vi "Custom Drive Motors.vi"(8 "error in (no error)":errorcluster, 9 "RightSpeed":dbl, 10 "LeftSpeed":dbl, 11 "RobotDriveDevRef":T1={"DevStatus"={"status"=FALSE, "code"=0, "source"=""}, "Motors[]"=[], "Square Inputs"=FALSE, "Max Output"=1.0}) -> (0 "error out":errorcluster, 2 "Motor Values":dbl[](array[numeric]), 3 "RobotDriveDevRef":T1={"DevStatus"={"status"=FALSE, "code"=0, "source"=""}, "Motors[]"=[], "Square Inputs"=FALSE, "Max Output"=1.0})   [LabVIEW 2015]
doc: "Determines the motor configuration and sends the speed values to the appropriate motors.\n\nThis software is licensed. Open the labview\\readme\\WPI Robotics Library Open Source License.txt file for more information."
uses:
  <vilib>/Rock Robotics/WPI/RobotDrive/WPI_RobotDriveDevRef.ctl
  <vilib>/Rock Robotics/WPI/MotorControl/WPI_MotorControlDeviceRef.ctl
  <vilib>/Rock Robotics/WPI/MotorControl/WPI_MotorControlType.ctl
  <vilib>/Rock Robotics/SystemInterfaces/DIO/FPGA_DIOPWMChannel.ctl
  <vilib>/Rock Robotics/WPI/PWM/WPI_PWMDeadband.ctl
  <vilib>/Rock Robotics/WPI/CAN/Jaguar/SubVIs/WPI_CANJaguar_ControlMode.ctl
  <vilib>/Rock Robotics/WPI/CAN/TalonSRX/WPI_CANTalonSRX_APIControlMode.ctl
  <vilib>/Rock Robotics/WPI/RobotDrive/WPI_RobotDriveSafetyCheck.vi
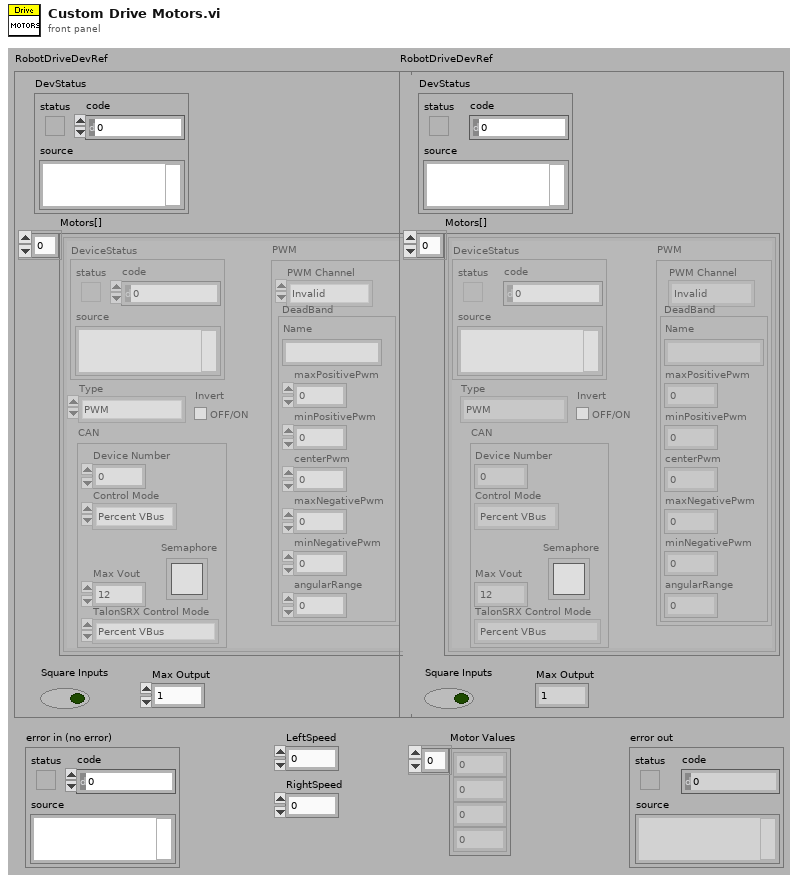
[diagram p1: front panel]
types:
  T1 = typedef "WPI_RobotDriveDevRef.ctl" = cluster{"DevStatus":errorcluster, "Motors[]":T2[], "Square Inputs":bool, "Max Output":dbl}
  T2 = typedef "WPI_MotorControlDeviceRef.ctl" = cluster{"DeviceStatus":errorcluster, "Type":T3, "PWM":cluster{"PWM Channel":T4, "DeadBand":T5}, "CAN":cluster{"Device Number":u8, "Control Mode":T6, "Semaphore":T7, "Max Vout":dbl, "TalonSRX Control Mode":T8}, "Invert":bool}
  T3 = typedef "WPI_MotorControlType.ctl" = enum16{"PWM", "CAN", "CANTalonSRX"}
  T4 = typedef "FPGA_DIOPWMChannel.ctl" = enum8{"PWM 0", "PWM 1", "PWM 2", "PWM 3", "PWM 4", "PWM 5", "PWM 6", "PWM 7", "PWM 8", "PWM 9", "PWM MXP 0", "PWM MXP 1", "PWM MXP 2", "PWM MXP 3", "PWM MXP 4", "PWM MXP 5", "PWM MXP 6", "PWM MXP 7", "PWM MXP 8", "PWM MXP 9", "Invalid"}
  T5 = typedef "WPI_PWMDeadband.ctl" = cluster{"Name":string, "maxPositivePwm":i32, "minPositivePwm":i32, "centerPwm":i32, "maxNegativePwm":i32, "minNegativePwm":i32, "angularRange":u16}
  T6 = typedef "WPI_CANJaguar_ControlMode.ctl" = enum8{"Percent VBus", "Current", "Speed", "Position", "Voltage"}
  T7 = typedef "Semaphore RefNum" = refnum<k1>
  T8 = typedef "WPI_CANTalonSRX_APIControlMode.ctl" = enum8{"Percent VBus", "Speed", "Position", "Slave", "Unchanged / Invalid", "Voltage Compensation", "Current", "Motion Profile"}
  T9 = enum16{"Rear Left Motor", "Rear Right Motor", "Front Left Motor", "Front Right Motor", "Middle Right Motor", "Middle Left Motor"}
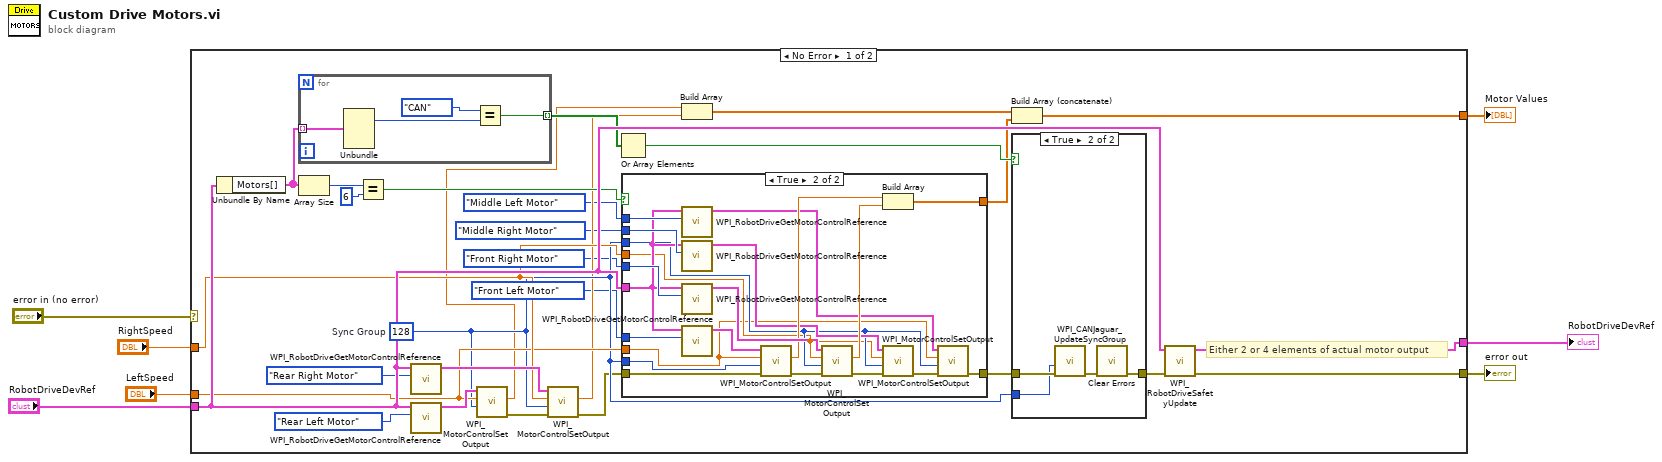
[diagram p0: block diagram]
diagram:
  n1 = case shown="No Error" "error in (no error)" {
    selector: "error in (no error)" -> [_ w69]
    tunnel: "RobotDriveDevRef" -> [w32 w68]
    tunnel: [w14 w68] -> w6
    tunnel: "LeftSpeed" -> [w30 _]
    tunnel: "RightSpeed" -> [w31 _]
    tunnel: [w15 w69] -> w2
    tunnel: [w17 _] -> w1
    frame No Error {
      w28 = u8 128  # Sync Group
      # "Either 2 or 4 elements of actual motor output"
      n2 = Unbundle By Name(w32) -> ("Motors[]"=w27:T2[])
      n3 = for {
        tunnel: w27 -> [w40] mode=indexing
        tunnel: [w37] -> w26 mode=indexing
        n4 = Unbundle(w40) -> ("Type"=w39:T3)  [unwired: 4 out]
        n5 = Equal?(x=enum16{"PWM", "CAN"}."CAN" ("Type"), y=w39) -> (x = y?=w37:bool)
      }
      n6 = Array Size(array=w27) -> (size(s)=w36:i32)
      n7 = Equal?(x=w36, y=6) -> (x = y?=w29:bool)
      n8 = call <vilib>:"WPI_RobotDriveGetMotorControlReference.vi"("MotorIndex"=T9."Rear Right Motor", "RobotDriveDevRef"=w32) -> ("MotorControlDeviceRef"=w34:T2)  [unwired: 9 out]
      n9 = call <vilib>:"WPI_RobotDriveGetMotorControlReference.vi"("MotorIndex"=T9."Rear Left Motor", "RobotDriveDevRef"=w32) -> ("MotorControlDeviceRef"=w33:T2)  [unwired: 9 out]
      n10 = call <vilib>:"WPI_MotorControlSetOutput.vi"("Sync Group / Parameter Slot"=w28, "Output"=w30, "MotorControlDevRef"=w33) -> ("error out"=w24:errorcluster, "Motor Output"=w21:dbl)  [unwired: 2 in, 5 out]
      n11 = call <vilib>:"WPI_MotorControlSetOutput.vi"("error in (no error)"=w24, "Sync Group / Parameter Slot"=w28, "Output"=w31, "MotorControlDevRef"=w34) -> ("error out"=w22:errorcluster, "Motor Output"=w20:dbl)  [unwired: 1 in, 5 out]
      n12 = Or Array Elements(Boolean array=w26) -> (logical OR=w25:bool)
      n13 = case shown="True" w29 {
        tunnel: T9."Front Left Motor" -> [_ w67]
        tunnel: T9."Front Right Motor" -> [_ w66]
        tunnel: w32 -> [_ w53]
        tunnel: w28 -> [_ w52]
        tunnel: w31 -> [_ w51]
        tunnel: w30 -> [_ w50]
        tunnel: [w46 w47] -> w23
        tunnel: w28 -> [_ w63]
        tunnel: w22 -> [w46 w61]
        tunnel: [_ w58] -> w19
        tunnel: T9."Middle Right Motor" -> [_ w56]
        tunnel: T9."Middle Left Motor" -> [_ w55]
        frame False {
        }
        frame True {
          n14 = call <vilib>:"WPI_RobotDriveGetMotorControlReference.vi"("MotorIndex"=w55, "RobotDriveDevRef"=w53) -> ("MotorControlDeviceRef"=w54:T2)  [unwired: 9 out]
          n15 = call <vilib>:"WPI_RobotDriveGetMotorControlReference.vi"("MotorIndex"=w56, "RobotDriveDevRef"=w53) -> ("MotorControlDeviceRef"=w57:T2)  [unwired: 9 out]
          n16 = call <vilib>:"WPI_RobotDriveGetMotorControlReference.vi"("MotorIndex"=w66, "RobotDriveDevRef"=w53) -> ("MotorControlDeviceRef"=w65:T2)  [unwired: 9 out]
          n17 = call <vilib>:"WPI_RobotDriveGetMotorControlReference.vi"("MotorIndex"=w67, "RobotDriveDevRef"=w53) -> ("MotorControlDeviceRef"=w64:T2)  [unwired: 9 out]
          n18 = call <vilib>:"WPI_MotorControlSetOutput.vi"("error in (no error)"=w61, "Sync Group / Parameter Slot"=w63, "Output"=w50, "MotorControlDevRef"=w64) -> ("error out"=w62:errorcluster, "Motor Output"=w59:dbl)  [unwired: 1 in, 5 out]
          n19 = call <vilib>:"WPI_MotorControlSetOutput.vi"("error in (no error)"=w62, "Sync Group / Parameter Slot"=w52, "Output"=w51, "MotorControlDevRef"=w65) -> ("error out"=w49:errorcluster, "Motor Output"=w60:dbl)  [unwired: 1 in, 5 out]
          n20 = Build Array(w59, w60) -> (w58:dbl[])
          n21 = call <vilib>:"WPI_MotorControlSetOutput.vi"("error in (no error)"=w49, "Sync Group / Parameter Slot"=w52, "Output"=w51, "MotorControlDevRef"=w57) -> ("error out"=w48:errorcluster)  [unwired: 1 in, 6 out]
          n22 = call <vilib>:"WPI_MotorControlSetOutput.vi"("error in (no error)"=w48, "Sync Group / Parameter Slot"=w52, "Output"=w50, "MotorControlDevRef"=w54) -> ("error out"=w47:errorcluster)  [unwired: 1 in, 6 out]
        }
      }
      n23 = Build Array(w21, w20) -> (w18:dbl[])
      n24 = Build Array (concatenate)(w18, w19) -> (w17:dbl[])
      n25 = case shown="True" w25 {
        tunnel: w23 -> [w41 w44]
        tunnel: w28 -> [_ w43]
        tunnel: [w41 w42] -> w16
        frame False {
        }
        frame True {
          n26 = call <vilib>:"WPI_CANJaguar_UpdateSyncGroup.vi"("error in (no error)"=w44, "Sync Group"=w43) -> ("error out"=w45:errorcluster)  [unwired: 9 out]
          n27 = call <vilib>:"Clear Errors.vi"("error in (no error)"=w45) -> ("error out"=w42:errorcluster)  [unwired: 1 in, 5 out]
        }
      }
      n28 = call <vilib>:"WPI_RobotDriveSafetyUpdate.vi"("error in (no error)"=w16, "RobotDriveDevRef"=w32) -> ("error out"=w15:errorcluster, "RobotDriveDevRef"=w14:T1)  [unwired: 8 out]
    }
    frame Error {
    }
  }
  "RobotDriveDevRef" <- w6
  "error out" <- w2
  "Motor Values" <- w1
